vi "Base Inject Alone.vi"(8 "P2 Disp Speed":dbl=5.0, 9 "P2 Asp Speed":dbl=20.0, 10 "NaOH Steps":u32=400) -> ()   [LabVIEW 2013]
uses:
  <vilib>/FPGAPlugInAG/sbRIO-9642/niLvFpga_Open_sbRIO-9642.vi
  <vilib>/rvi/interface/common/dynamic/niFpgaDynamicAddResources.vi
  <vilib>/rvi/interface/common/niFpgaWaitOnOcc.vi
  <vilib>/Utility/error.llb/Error Cluster From Error Code.vi
  <vilib>/rvi/errors/niLvFpgaAdjustHostInterfaceError.vi
  <vilib>/FPGAPlugInAG/Dynamic/niLvFpga_Close_Dynamic.vi
  <vilib>/rvi/interface/nirviOpenFPGA/nirviOpenFPGA.xnode
  FPGA Bitfiles/TCO2DeploymentPr_FPGATarget_FullyLoadedFPGA_JLaDFRu0zCY.lvbitx
  FPGA Code/Fully Loaded FPGA.vi
  <vilib>/rvi/interface/nirviReadWriteControl/nirviReadWriteControl.xnode
  <vilib>/rvi/interface/nirviCloseFPGA/nirviCloseFPGA.xnode
  <vilib>/rvi/interface/Simulation/niFpgaSimulationCallBeginRW.vi
  NiFpgaLv.dll
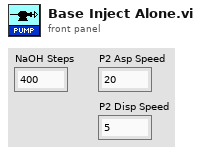
[diagram p1: front panel]
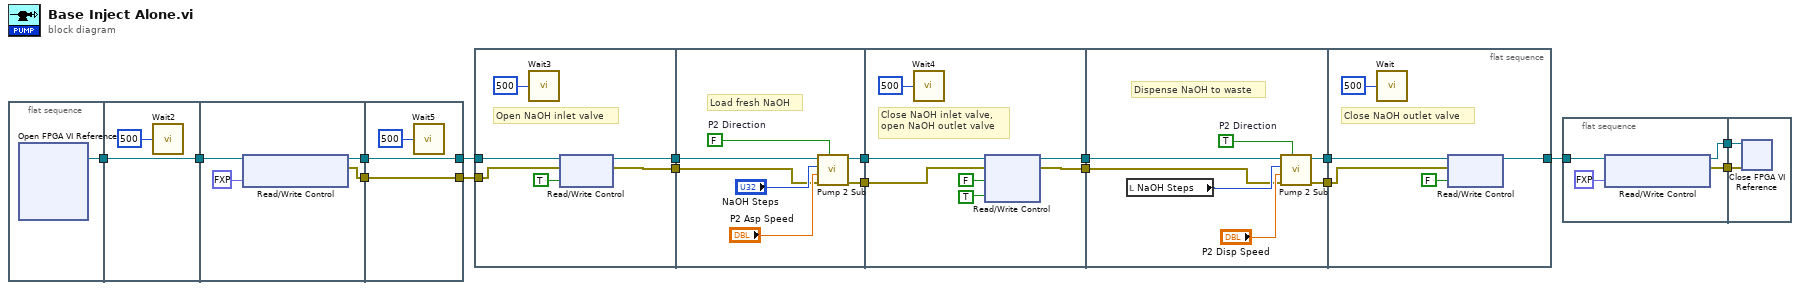
[diagram p0: block diagram]
diagram:
  n1 = flat-sequence {
    tunnel: [w18] -> w17
    tunnel: w17 -> [w20]
    tunnel: [w20] -> w16
    tunnel: w16 -> [w24]
    tunnel: [w23] -> w15
    tunnel: [w21] -> w3
    tunnel: w15 -> [w26]
    tunnel: [w26] -> w14
    tunnel: [w25] -> w4
    tunnel: w3 -> [w25]
    frame #0 {
      n2 = xnode "Open FPGA VI Reference"() -> ("FPGA VI Reference Out"=w18:refnum<k20>)  [unwired: 2 in, 1 out]
    }
    frame #1 {
      n3 = call "Wait2"("Count(mSec)"=u32 500) -> ()  [unwired: 1 out]
    }
    frame #2 {
      n4 = xnode "Read/Write Control"("FPGA VI Reference In"=w24, "SwitchP (10=on)"=fxp<+/-,20,5> 10.0) -> ("FPGA VI Reference Out"=w23:refnum<k20>, "error out"=w21:errorcluster)  [unwired: 1 in]
    }
    frame #3 {
      n5 = call "Wait5"("Count(mSec)"=u32 500) -> ()  [unwired: 1 out]
    }
  }
  n6 = flat-sequence {
    tunnel: w14 -> [w31]
    tunnel: [w30] -> w10
    tunnel: [w29] -> w5
    tunnel: w4 -> [w28]
    tunnel: w10 -> [w37]
    tunnel: [w36] -> w9
    tunnel: [w35] -> w6
    tunnel: w5 -> [w34]
    tunnel: w9 -> [w44]
    tunnel: [w43] -> w8
    tunnel: [w42] -> w7
    tunnel: w6 -> [w41]
    tunnel: w8 -> [w51]
    tunnel: w7 -> [w50]
    tunnel: [w49] -> w2
    tunnel: [w48] -> w1
    tunnel: [w59] -> w11
    tunnel: w2 -> [w56]
    tunnel: w1 -> [w55]
    frame #0 {
      # "Open NaOH inlet valve"
      n7 = call "Wait3"("Count(mSec)"=u32 500) -> ()  [unwired: 1 out]
      n8 = xnode "Read/Write Control"("FPGA VI Reference In"=w31, "error in"=w28, "VBAsp"=TRUE ("V2-P1 Waste")) -> ("FPGA VI Reference Out"=w30:refnum<k20>, "error out"=w29:errorcluster)
    }
    frame #1 {
      w40 = FALSE  # P2 Direction
      # "Load fresh NaOH"
      n9 = call "Pump 2 Sub.vi"("P2 Direction"=w40, "Error In"=w34, "P2 pps"="P2 Asp Speed", "P2 Steps"="NaOH Steps", "FPGA ref in"=w37) -> ("Error out"=w35:errorcluster, "FPGA ref out"=w36:refnum<k20>)  [unwired: 5 in]
    }
    frame #2 {
      # "Close NaOH inlet valve, \nopen NaOH outlet valve"
      n10 = call "Wait4"("Count(mSec)"=u32 500) -> ()  [unwired: 1 out]
      n11 = xnode "Read/Write Control"("FPGA VI Reference In"=w44, "error in"=w41, "VBAsp"=FALSE ("V1-Acid"), "VBDisp"=TRUE ("V2-P1 Waste")) -> ("FPGA VI Reference Out"=w43:refnum<k20>, "error out"=w42:errorcluster)
    }
    frame #3 {
      w54 = TRUE  # P2 Direction
      # "Dispense NaOH to waste"
      n12 = local read "NaOH Steps"() -> (w52:u32)
      n13 = call "Pump 2 Sub.vi"("P2 Direction"=w54, "Error In"=w50, "P2 pps"="P2 Disp Speed", "P2 Steps"=w52, "FPGA ref in"=w51) -> ("Error out"=w48:errorcluster, "FPGA ref out"=w49:refnum<k20>)  [unwired: 5 in]
    }
    frame #4 {
      # "Close NaOH outlet valve"
      n14 = call "Wait"("Count(mSec)"=u32 500) -> ()  [unwired: 1 out]
      n15 = xnode "Read/Write Control"("FPGA VI Reference In"=w56, "error in"=w55, "VBDisp"=FALSE ("V4-P2 Waste")) -> ("FPGA VI Reference Out"=w59:refnum<k20>)  [unwired: 1 out]
    }
  }
  n16 = flat-sequence {
    tunnel: [w63] -> w13
    tunnel: [w62] -> w12
    tunnel: w11 -> [w60]
    tunnel: w13 -> [w65]
    tunnel: w12 -> [w64]
    frame #0 {
      n17 = xnode "Read/Write Control"("FPGA VI Reference In"=w60, "SwitchP (10=on)"=fxp<+/-,20,5> 0.0) -> ("FPGA VI Reference Out"=w63:refnum<k20>, "error out"=w62:errorcluster)  [unwired: 1 in]
    }
    frame #1 {
      n18 = xnode "Close FPGA VI Reference"("FPGA VI Reference In"=w65, "error in"=w64) -> ()  [unwired: 1 out]
    }
  }
